vi "Plot_RoofShape.vi"() -> ()   [LabVIEW 2014]
uses:
  Anemometry/Anemometry Sub Vis/Controls/Server_Comms.ctl
  Anemometry/Anemometry Sub Vis/File/Setup_Filetype.ctl
  <vilib>/printing/EasyPrintingControls.llb/report_type.ctl
  <vilib>/printing/EasyPrintingControls.llb/layout_options.ctl
  <vilib>/printing/EasyPrintingControls.llb/orientation.ctl
  <vilib>/printing/EasyPrintingControls.llb/panel_scaling_for_page.ctl
  <vilib>/printing/EasyPrintingControls.llb/margins.ctl
  <vilib>/printing/EasyPrintingControls.llb/margin_values.ctl
  <vilib>/printing/EasyPrintingControls.llb/measurement_system.ctl
  <vilib>/printing/EasyPrintingControls.llb/printer_options.ctl
  <vilib>/printing/EasyPrintingControls.llb/printing_method.ctl
  <vilib>/printing/EasyPrintingControls.llb/color_or_monochrome.ctl
  <vilib>/printing/EasyPrintingControls.llb/page_header_options.ctl
  <vilib>/printing/EasyPrintingControls.llb/page_headers.ctl
  <vilib>/printing/EasyPrintingControls.llb/page_header_content_options.ctl
  <vilib>/printing/EasyPrintingControls.llb/custom_contents_options.ctl
  <vilib>/printing/EasyPrintingControls.llb/list_which_controls.ctl
  Anemometry/Anemometry Sub Vis/Globals/Preference_global.vi
  <vilib>/printing/EasyPrinting.llb/Easy Print VI Panel or Documentation (path).vi
  <vilib>/Utility/NIReport.llb/NI_ReportGenerationCore.lvlib
  <vilib>/Utility/SMTP/NI_SMTPEmail.lvlib
panel:
  in  "Units Selector":u16(ring) items=["Metric", "English"]
  in  "Tab Control":T1(tab)=enum."Real-Time"
  in  "History\n(mins)":dbl=2.0 format="%.1f"
  in  "Mode":T2(ring)=enum."Display data over specified period:"
  in  "Throwback\n(mins)":dbl format="%.1f"
  out "LastUpdated":string="Wed, Jul 29, 2015 at 4:31 PM"
  out "Plot 1":cluster{"Times":dbl[], "Output array":dbl[]}[](graph)
  in  "Search 4":string="tunnel3:avstat" caption="Search:"
  in  "Selector 4":i32[](listbox)=[0, 1, 2, 3, 4, 5, 6, 7, 8, 9]
  in  "Save 1":bool
  in  "Precision":i32=2
  in  "Selector 5":i32[](listbox)=[0, 1, 2, 3, 4, 5, 6, 7]
  in  "Search 5":string="tunnel3:Avstat" caption="Search:"
  in  "Selector 6":i32[](listbox)=[0, 1, 2, 3, 4, 5, 6, 7]
  in  "Search 6":string="rangeroof" caption="Search:"
  out "x < y?":bool=TRUE caption="In Range"
  in  "Save 3":bool
  out "Plot 3":cluster{"Times":dbl[], "Output array":dbl[]}[](graph)=[{"Times"=[1.0, 2.0, 3.0, 4.0, 5.0, 6.0, 7.0, 8.0], "Output array"=[0.0, 0.0, 0.0, 4.0, 9.0, 11.0, 13.0, 3.0]}, {"Times"=[1.0, 2.0, 3.0, 4.0, 5.0, 6.0, 7.0, 8.0], "Output array"=[-0.002410980854964788, -0.0029939228778896234, -0.002989543855604076, -0.000737475319318735, -0.0014917557433837283, -0.0018513430195620808, -0.0021749907541396205, -0.0013073221118501653]}, {"Times"=[8.0, 1.0], "Output array"=[-0.000737475319318735, -0.000737475319318735]}, {"Times"=[8.0, 1.0], "Output array"=[-0.0029939228778896234, -0.0029939228778896234]}]
  out "Roof Height":dbl[](array[numeric])=[0.0, 0.0, 0.0, 4.0, 9.0, 11.0, 13.0, 3.0] caption="Roof Height (cm)"
  out "Failed recipients":string[](array[string])
  in  "Recipients":string[](array[string])=["ttech@cppwind.com"]
  in  "mail server":string="post.cppwind.local"
  in  "print?":bool
  in  "email?":bool
  in  "Save plot number":T3(ring)
  out "Plot 1 Chs":string[](array[string])=["Tunnel3:AvStat:P1", "Tunnel3:AvStat:P2", "Tunnel3:AvStat:P3", "Tunnel3:AvStat:P4", "Tunnel3:AvStat:P5", "Tunnel3:AvStat:P6", "Tunnel3:AvStat:P7", "Tunnel3:AvStat:P8", "Tunnel3:AvStat:+PFan", "Tunnel3:AvStat:P0"]
  out "Plot 2 Chs":string[](array[string])=["Tunnel3:AvStat:P1", "Tunnel3:AvStat:P2", "Tunnel3:AvStat:P3", "Tunnel3:AvStat:P4", "Tunnel3:AvStat:P5", "Tunnel3:AvStat:P6", "Tunnel3:AvStat:P7", "Tunnel3:AvStat:P8"]
  out "Plot 3 Chs":string[](array[string])=["Tunnel3:RangeRoof:1", "Tunnel3:RangeRoof:2", "Tunnel3:RangeRoof:3", "Tunnel3:RangeRoof:4", "Tunnel3:RangeRoof:5", "Tunnel3:RangeRoof:6", "Tunnel3:RangeRoof:7", "Tunnel3:RangeRoof:8"]
  in  "Save 2":bool
  out "Plot 2":cluster{dbl[], "Output array":dbl[]}(graph)={[1.0, 2.0, 3.0, 4.0, 5.0, 6.0, 7.0, 8.0], "Output array"=[-0.002410980854964788, -0.0029939228778896234, -0.002989543855604076, -0.000737475319318735, -0.0014917557433837283, -0.0018513430195620808, -0.0021749907541396205, -0.0013073221118501653]}
  in  "stop":bool=TRUE
  # "Select Pressure Measurement"
  # "Select Height Measurement"
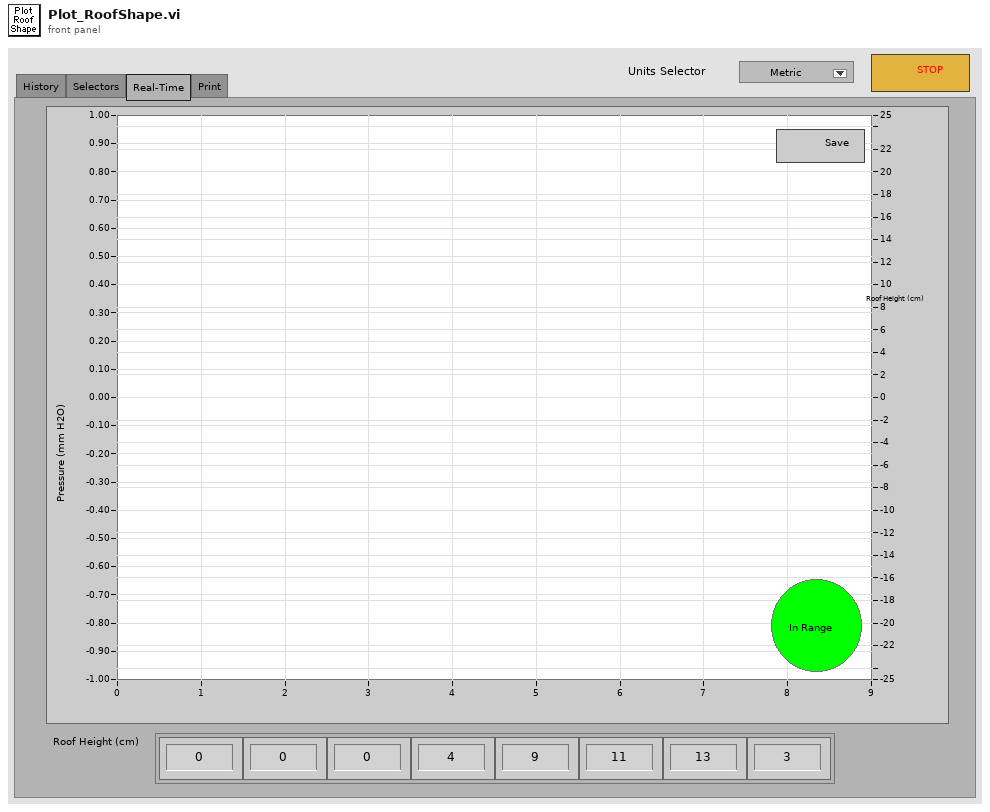
[diagram p1: front panel]
types:
  T1 = enum32{"History", "Selectors", "Real-Time", "Print"}
  T2 = enum16{"Display full time history", "Display data over specified period:"}
  T3 = enum16{"Save Plot 1", "Save Plot 2", "Save Plot 3"}
  T4 = typedef "Server_Comms.ctl" = enum16{"Server Link Healthy", "Do Not Link To Server"}
  T5 = typedef "Setup_Filetype.ctl" = enum16{"Measurement Setups", "Calibration Setups", "General", "Results File Plotter Setups", "Speed Calib Tweaks"}
  T6 = cluster{"path":path, "data":string, "binary":bool, "MIME content-type \n(application/octet-stream)":string}
  T7 = typedef "NI_ReportGenerationCore.lvlib/custom_contents_options.ctl" = cluster{"include VI connector and icon":bool, "include VI description":bool, "include front panel":bool, "surround front panel with border":bool, "list of controls options":cluster{"include list of controls":bool, "list which controls?":T8, "include control descriptions?":bool, "include control data types?":bool}, "block diagram options":cluster{"include block diagram":bool, "hidden frames":bool, "ordered (repeat from higher level if nested)":bool}, "include VI hierarchy":bool, "include list of subVIs":bool, "include VI history":bool, "include Express VI configuration information":bool}
  T8 = typedef "NI_ReportGenerationCore.lvlib/list_which_controls.ctl" = u16
  T9 = typedef "NI_ReportGenerationCore.lvlib/layout_options.ctl" = cluster{"orientation (unchanged)":T10, "panel scaling for page (unchanged)":T11, "margins":T12, "printer options":T15, "page header options":T18}
  T10 = typedef "NI_ReportGenerationCore.lvlib/orientation.ctl" = u16
  T11 = typedef "NI_ReportGenerationCore.lvlib/panel_scaling_for_page.ctl" = u16
  T12 = typedef "NI_ReportGenerationCore.lvlib/margins.ctl" = cluster{"override VI margins (false)":bool, "margins (1.00)":T13, "measurement system (default)":T14}
  T13 = typedef "NI_ReportGenerationCore.lvlib/margin_values.ctl" = cluster{"top":dbl, "left":dbl, "right":dbl, "bottom":dbl}
  T14 = typedef "NI_ReportGenerationCore.lvlib/measurement_system.ctl" = u16
  T15 = typedef "NI_ReportGenerationCore.lvlib/printer_options.ctl" = cluster{"destination printer name (current)":string, "printing method (unchanged)":T16, "color or monochrome (unchanged)":T17}
  T16 = typedef "NI_ReportGenerationCore.lvlib/printing_method.ctl" = u16
  T17 = typedef "NI_ReportGenerationCore.lvlib/color_or_monochrome.ctl" = u16
  T18 = typedef "NI_ReportGenerationCore.lvlib/page_header_options.ctl" = cluster{"page headers (unchanged)":T19, "page header content options":T20}
  T19 = typedef "NI_ReportGenerationCore.lvlib/page_headers.ctl" = u16
  T20 = typedef "NI_ReportGenerationCore.lvlib/page_header_content_options.ctl" = cluster{"Include VI Name":bool, "Include VI Path":bool, "Include Last Modification Date":bool, "Include Date Printed":bool, "Include Page Number":bool, "Include VI Icon":bool}
  T21 = typedef "NI_ReportGenerationCore.lvlib/report_type.ctl" = u16
  T22 = cluster{"path":path, "data":string, "binary":bool, "MIME content-type \n(application/octet-stream)":string}[]
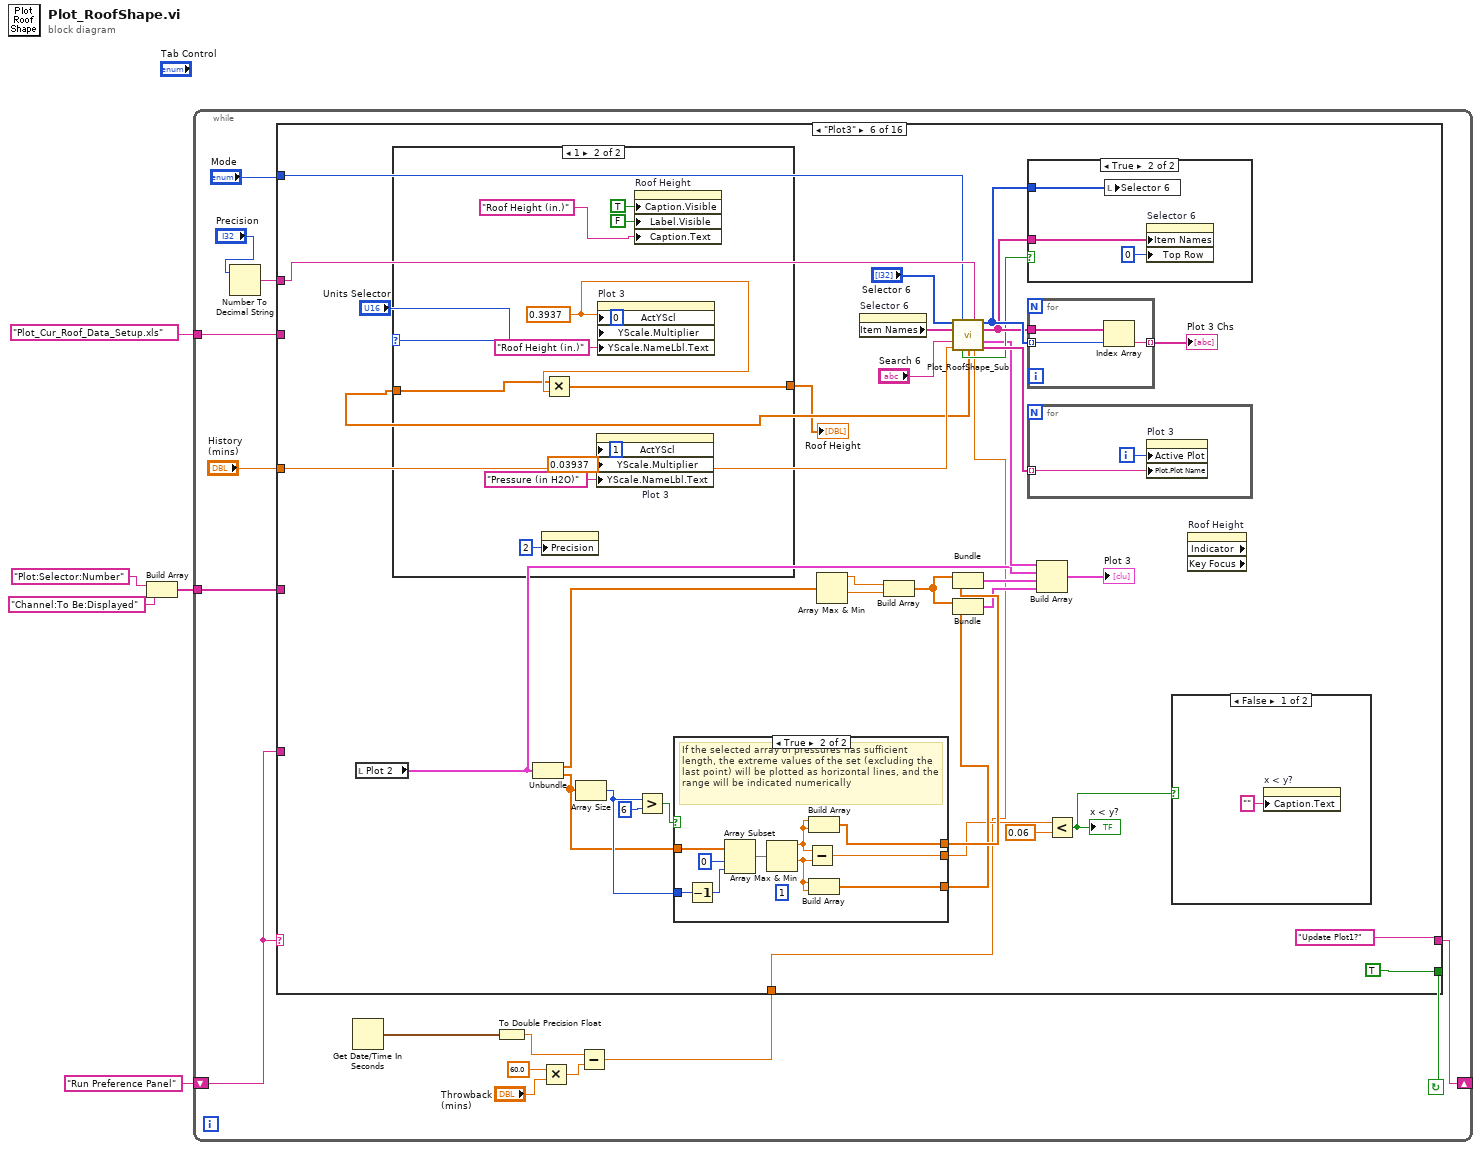
[diagram p0: block diagram]
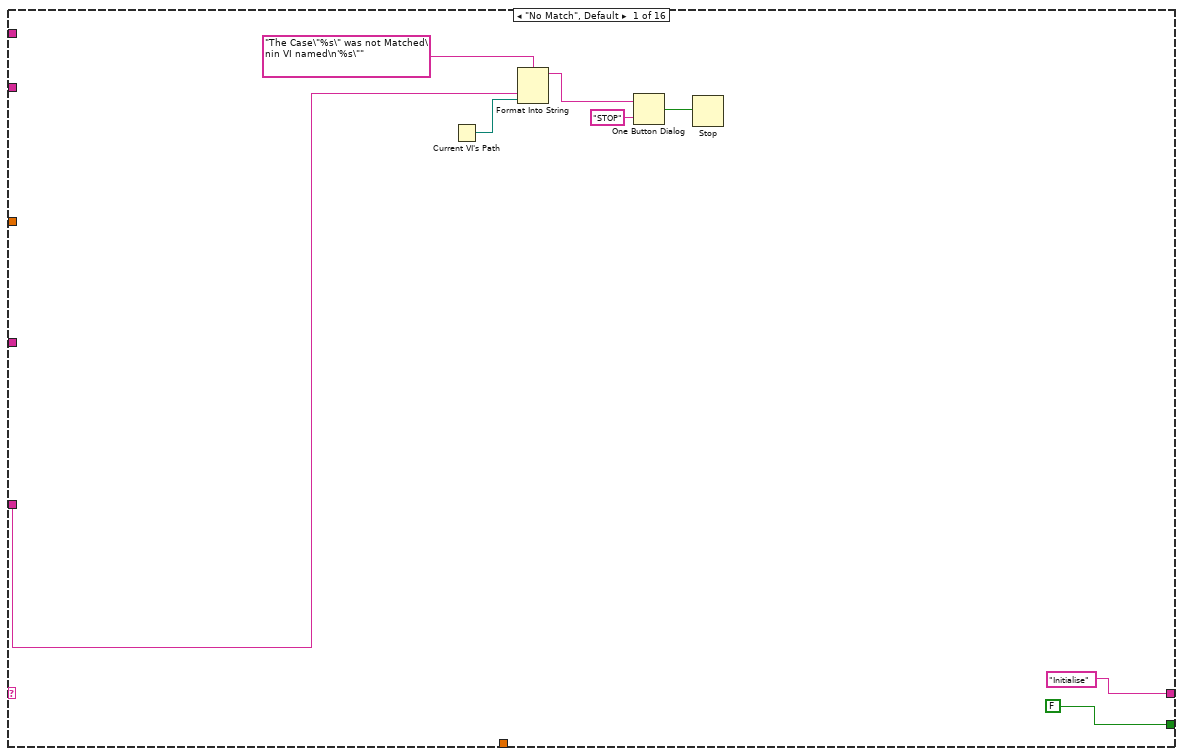
[diagram p2: hidden frame]
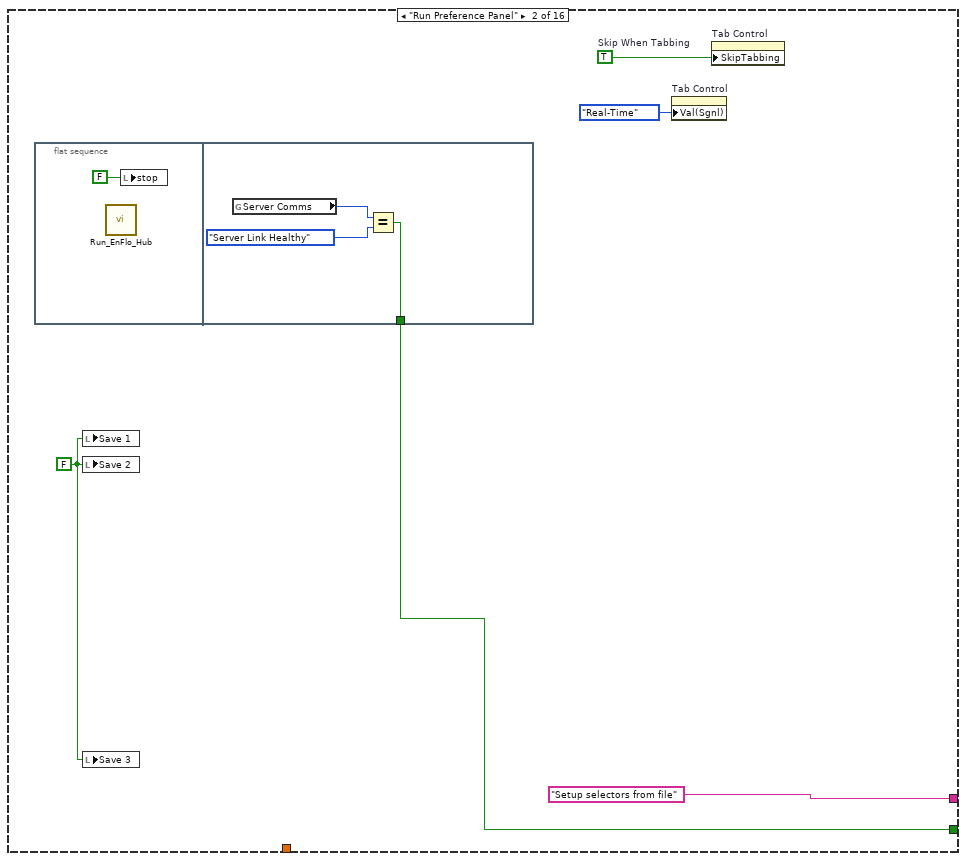
[diagram p3: hidden frame]
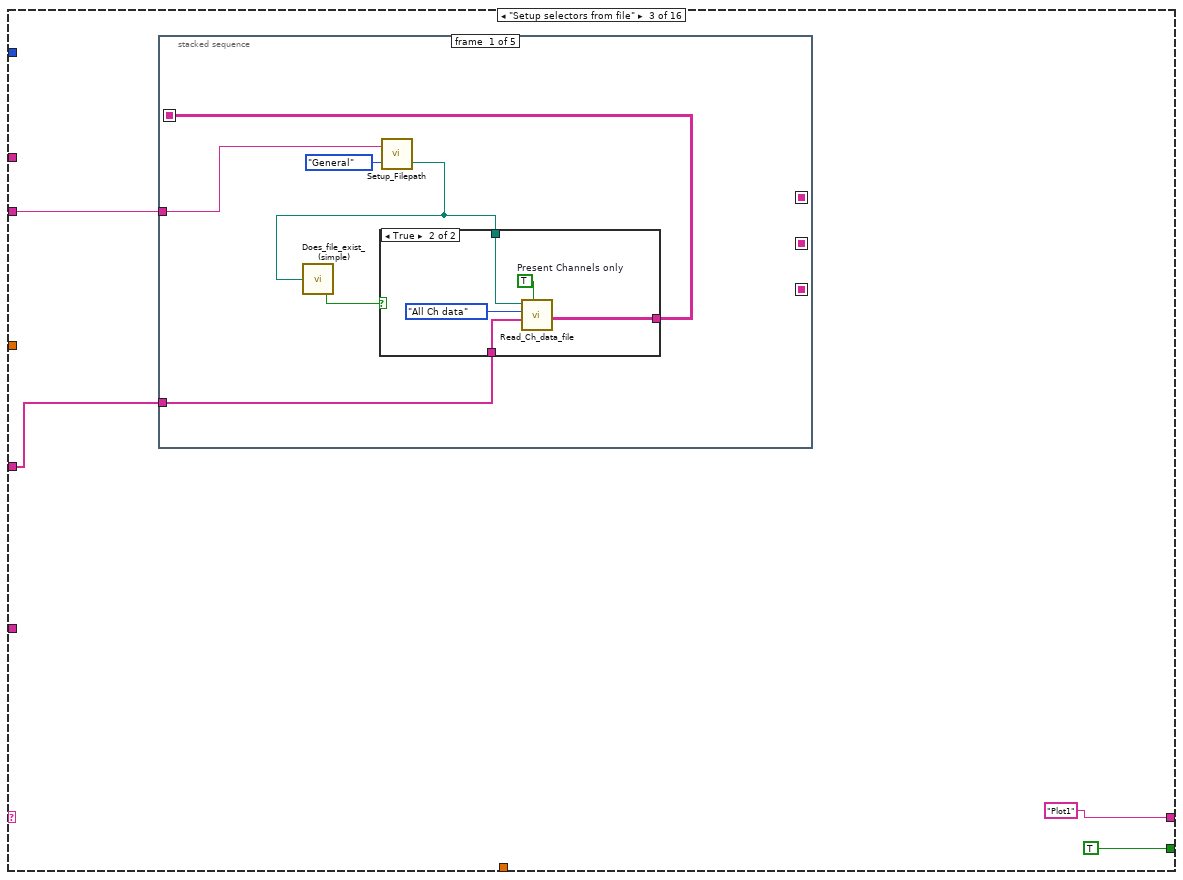
[diagram p4: hidden frame]
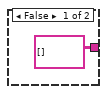
[diagram p5: hidden frame]
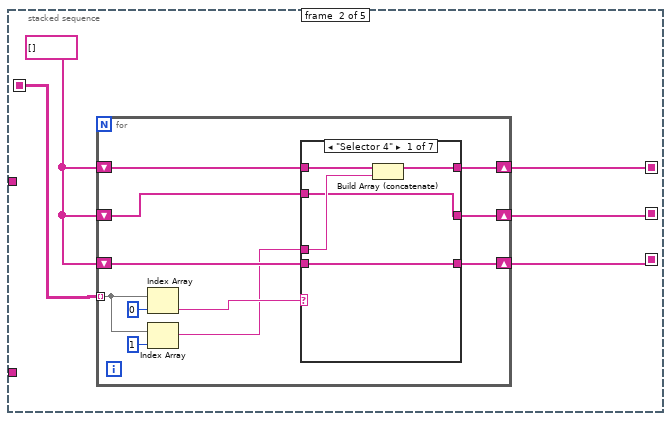
[diagram p6: hidden frame]
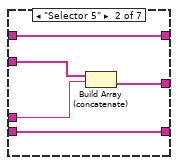
[diagram p7: hidden frame]
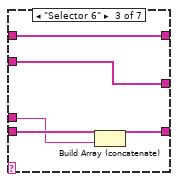
[diagram p8: hidden frame]
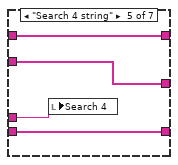
[diagram p10: hidden frame]
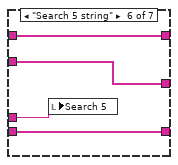
[diagram p11: hidden frame]
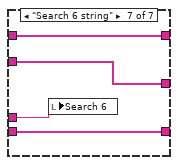
[diagram p12: hidden frame]
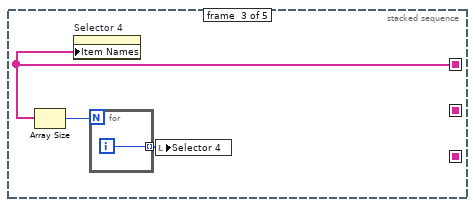
[diagram p13: hidden frame]
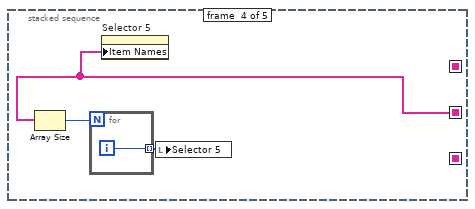
[diagram p14: hidden frame]
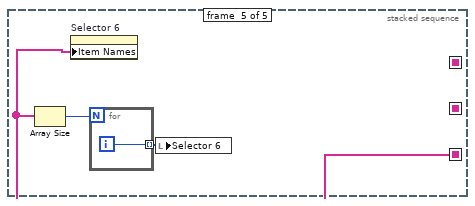
[diagram p15: hidden frame]
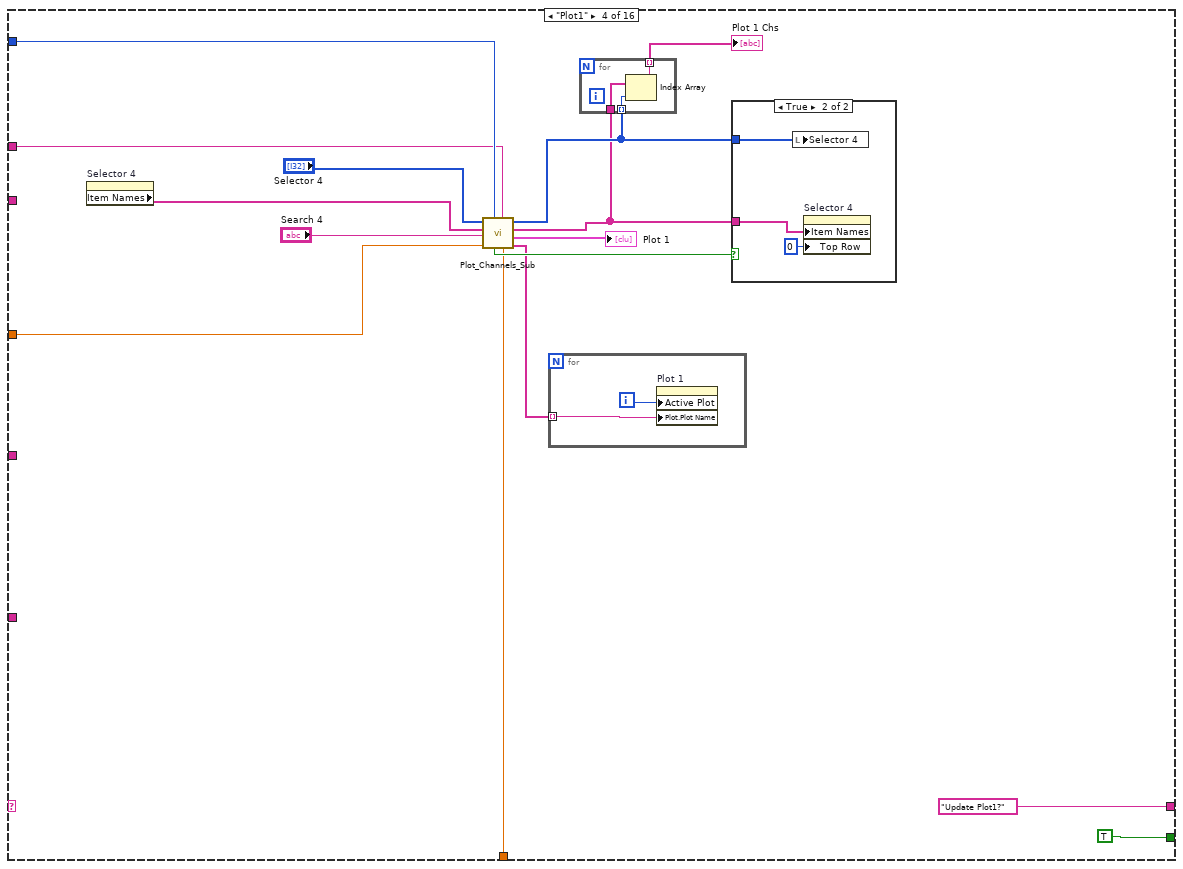
[diagram p16: hidden frame]
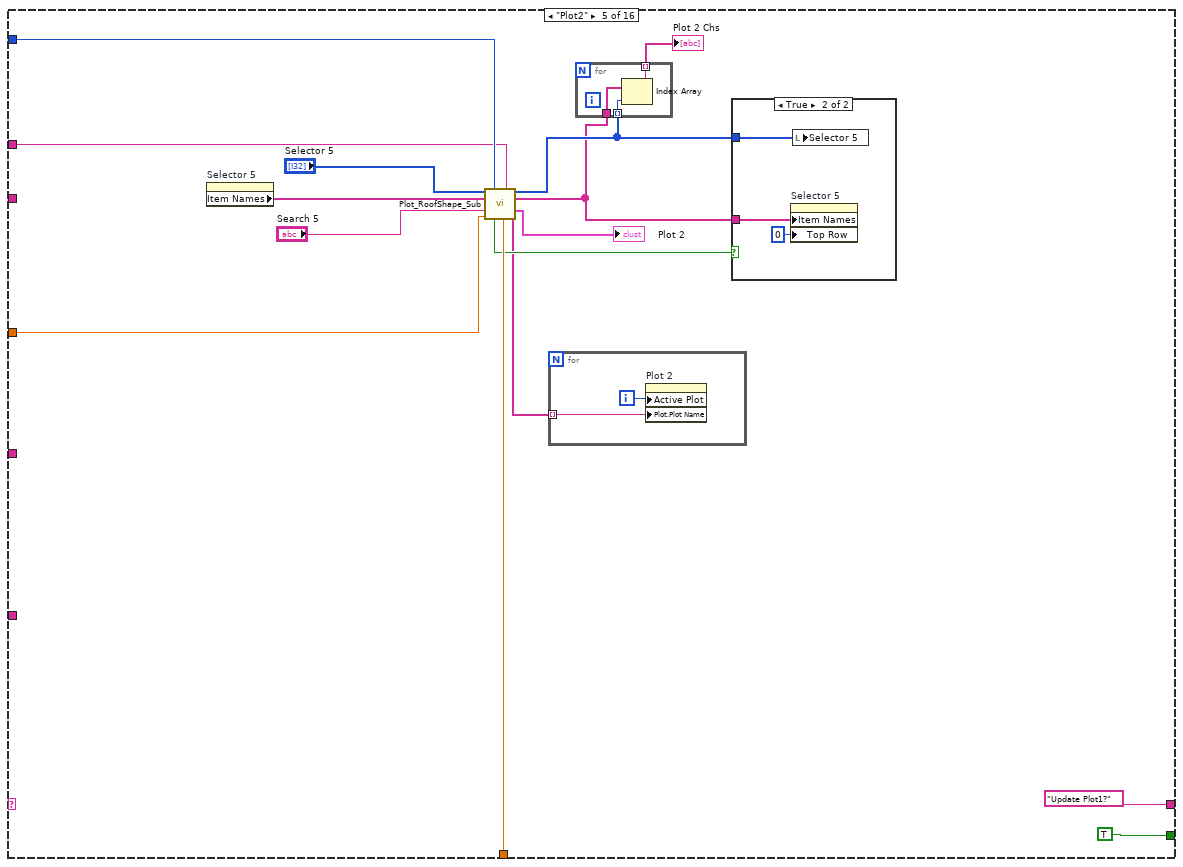
[diagram p18: hidden frame]
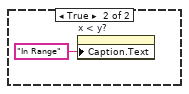
[diagram p20: hidden frame]
diagram:
  n1 = Build Array("Plot:Selector:Number", "Channel:To Be:Displayed") -> (w2:string[])
  n2 = while {
    shift-left: "Run Preference Panel" -> [w18]
    shift-right: [w19] -> _
    tunnel: w2 -> [w15]
    tunnel: "Plot_Cur_Roof_Data_Setup.xls" -> [w14]
    stop <- w20 continue-if-true
    n3 = Number To Decimal String(number="Precision") -> (decimal integer string=w12:string)  [unwired: 1 out]
    n4 = Get Date/Time In Seconds() -> (seconds since 1Jan1904=w11:timestamp)
    n5 = To Double Precision Float(number=w11) -> (double precision float=w7:dbl)
    n6 = Multiply(x=60.0, y="Throwback\n(mins)") -> (x*y=w8:dbl)
    n7 = Subtract(x=w7, y=w8) -> (x-y=w6:dbl)
    n8 = case shown="\"Plot3\"" w18 {
      tunnel: [FALSE w32 TRUE TRUE TRUE TRUE TRUE TRUE TRUE TRUE w371 TRUE TRUE TRUE TRUE w473] -> w20
      tunnel: ["Initialise" "Setup selectors from file" "Plot1" "Update Plot1?" "Update Plot1?" "Update Plot1?" w239 w260 w280 w300 w372 w431 "Email" ("t") "CleanUp" ("t") "What to do next?" "Update Plot1?" ("t")] -> w19
      tunnel: w18 -> [w23 _ _ _ _ _ _ _ _ _ _ _ _ _ _ _]
      tunnel: "Mode" -> [_ _ _ w119 w140 w180 _ _ _ _ _ _ _ _ _ _]
      tunnel: "History\n(mins)" -> [_ _ _ w118 w145 w189 _ _ _ _ _ _ _ _ _ _]
      tunnel: w15 -> [_ _ w38 _ _ _ _ _ _ _ _ _ _ _ _ w477]
      tunnel: w14 -> [_ _ w39 _ _ _ _ _ _ _ _ _ _ _ _ w476]
      tunnel: w12 -> [_ _ _ w113 w135 w185 _ _ _ _ _ _ _ _ _ _]
      tunnel: w6 -> [_ _ _ w112 w146 w162 _ _ _ _ _ _ _ _ _ _]
      frame "No Match", Default {
        n9 = Current VI's Path() -> (path=w22:path)
        n10 = Format Into String(format string="The Case\"%s\" was not Matched\nin VI named\n'%s\"" ("Format String"), w23, w22) -> (resulting string=w26:string)  [unwired: 2 in, 1 out]
        n11 = One Button Dialog(message=w26, button name ("OK")="STOP") -> (true=w24:bool)
        n12 = Stop(stop? (T)=w24) -> ()
      }
      frame "Run Preference Panel" {
        w29 = TRUE  # Skip When Tabbing
        w31 = FALSE ("Save 1")
        n13 = flat-sequence {
          tunnel: [w35] -> w32
          frame #0 {
            n14 = call "Run_EnFlo_Hub.vi"() -> ()  [unwired: 8 out]
            n15 = local write "stop"(FALSE ("stop")) -> ()
          }
          frame #1 {
            n16 = global read "Preference_global.vi" "Server Comms"() -> (w36:T4)
            n17 = Equal?(x=w36, y=Server_Comms."Server Link Healthy" ("Server Comms")) -> (x = y?=w35:bool)
          }
        }
        n18 = local write "Save 1"(w31) -> ()
        n19 = local write "Save 2"(w31) -> ()
        n20 = local write "Save 3"(w31) -> ()
        n21 = property on="Tab Control" class="TabCtl (strict)"("Val(Sgnl)"=T1."Real-Time" ("Value (Signaling)")) -> ()  [unwired: 2 in, 2 out]
        n22 = property on="Tab Control" class="TabCtl (strict)"("SkipTabbing"=w29) -> ()  [unwired: 2 in, 2 out]
      }
      frame "Setup selectors from file" {
        n23 = stacked-sequence {
          seq-local: [w45 _ _ _ _] -> [_ w58 _ _ _]
          seq-local: [_ w56 _ _ _] -> [_ _ w102 _ _]
          seq-local: [_ w54 _ _ _] -> [_ _ _ w104 _]
          seq-local: [_ w55 _ _ _] -> [_ _ _ _ w108]
          tunnel: w39 -> [w44 _ _ _ _]
          tunnel: w38 -> [w46 _ _ _ _]
          frame #0 {
            n24 = call "Setup_Filepath.vi"("Setup File Type"=Setup_Filetype."General", "Filename in"=w44) -> ("Filename Out"=w43:path)  [unwired: 1 out]
            n25 = call "Does_file_exist_(simple).vi"("Pathname"=w43) -> ("exists?"=w47:bool)
            n26 = case shown="True" w47 {
              tunnel: w43 -> [_ w53]
              tunnel: w46 -> [_ w52]
              tunnel: [string[][] [] ("Channel Values") w49] -> w45
              frame False {
              }
              frame True {
                w51 = TRUE  # Present Channels only
                n27 = call "Read_Ch_data_file.vi"("Present Channels only"=w51, "Present Channels"=w52, "Output"=enum16{"All Ch data", "The last few rows"}."All Ch data", "Filename"=w53) -> ("Channel Values"=w49:string[][])  [unwired: 1 in, 4 out]
              }
            }
          }
          frame #1 {
            w57 = string[] []
            n28 = for {
              shift-right: [w64] -> w56
              shift-left: w57 -> [w65]
              tunnel: w58 -> [w66] mode=indexing
              shift-right: [w62] -> w54
              shift-left: w57 -> [w63]
              shift-right: [w60] -> w55
              shift-left: w57 -> [w61]
              n29 = Index Array(array=w66, index=0 ("Index")) -> (element=w68:string)
              n30 = Index Array(array=w66, index=1 ("Index")) -> (element=w59:string)
              n31 = case shown="\"Selector 4\"" w68 {
                tunnel: w65 -> [w74 w79 w80 w86 w90 w94 w98]
                tunnel: [w73 w79 w80 w86 w90 w94 w98] -> w64
                tunnel: w59 -> [w72 w76 w82 _ w88 w92 w96]
                tunnel: w63 -> [w71 w77 w81 w87 w91 w95 w99]
                tunnel: [w71 w75 w81 w87 w91 w95 w99] -> w62
                tunnel: w61 -> [w70 w78 w84 w85 w89 w93 w97]
                tunnel: [w70 w78 w83 w85 w89 w93 w97] -> w60
                frame "Selector 4" {
                  n32 = Build Array (concatenate)(w74, w72) -> (w73:string[])
                }
                frame "Selector 5" {
                  n33 = Build Array (concatenate)(w77, w76) -> (w75:string[])
                }
                frame "Selector 6" {
                  n34 = Build Array (concatenate)(w84, w82) -> (w83:string[])
                }
                frame "No Match", Default {
                }
                frame "Search 4 string" {
                  n35 = local write "Search 4"(w88) -> ()
                }
                frame "Search 5 string" {
                  n36 = local write "Search 5"(w92) -> ()
                }
                frame "Search 6 string" {
                  n37 = local write "Search 6"(w96) -> ()
                }
              }
            }
          }
          frame #2 {
            n38 = Array Size(array=w102) -> (size(s)=w101:i32)
            n39 = property on="Selector 4" class="LstBox (strict)"("Item Names"=w102) -> ()  [unwired: 2 in, 2 out]
            n40 = for {
              N: w101 -> [_]
              tunnel: [w103] -> w100 mode=indexing
              i -> [w103]
            }
            n41 = local write "Selector 4"(w100) -> ()
          }
          frame #3 {
            n42 = Array Size(array=w104) -> (size(s)=w106:i32)
            n43 = for {
              N: w106 -> [_]
              tunnel: [w107] -> w105 mode=indexing
              i -> [w107]
            }
            n44 = property on="Selector 5" class="LstBox (strict)"("Item Names"=w104) -> ()  [unwired: 2 in, 2 out]
            n45 = local write "Selector 5"(w105) -> ()
          }
          frame #4 {
            n46 = Array Size(array=w108) -> (size(s)=w110:i32)
            n47 = property on="Selector 6" class="LstBox (strict)"("Item Names"=w108) -> ()  [unwired: 2 in, 2 out]
            n48 = for {
              N: w110 -> [_]
              tunnel: [w111] -> w109 mode=indexing
              i -> [w111]
            }
            n49 = local write "Selector 6"(w109) -> ()
          }
        }
      }
      frame "Plot1" {
        n50 = property on="Selector 4" class="LstBox (strict)"() -> ("Item Names"=w121:string[])  [unwired: 2 in, 2 out]
        n51 = call "Plot_Channels_Sub.vi"("End Time"=w112, "precision"=w113, "Mode"=w119, "History (min)"=w118, "Search String"="Search 4", "Selector List In"=w121, "Selector array In"="Selector 4") -> ("Plot Legend"=w117:string[], "Plot"=→"Plot 1":cluster{"Times":dbl[], "Output array":dbl[]}[], "Selector List Out"=w115:string[], "Selector array Out"=w116:i32[], "Selector Changed?"=w123:bool)
        n52 = for {
          tunnel: w117 -> [w130] mode=indexing
          i -> [w131]
          n53 = property on="Plot 1" class="XYGraph (strict)"("Active Plot"=w131, "Plot.Plot Name"=w130) -> ()  [unwired: 2 in, 2 out]
        }
        n54 = for {
          tunnel: w116 -> [w129] mode=indexing
          tunnel: w115 -> [w128]
          tunnel: [w127] -> w114 mode=indexing
          n55 = Index Array(array=w128, index=w129) -> (element=w127:string)
        }
        "Plot 1 Chs" <- w114
        n56 = case shown="True" w123 {
          tunnel: w115 -> [_ w134]
          tunnel: w116 -> [_ w133]
          frame False {
          }
          frame True {
            n57 = local write "Selector 4"(w133) -> ()
            n58 = property on="Selector 4" class="LstBox (strict)"("Item Names"=w134, "Top Row"=0) -> ()  [unwired: 2 in, 2 out]
          }
        }
      }
      frame "Plot2" {
        n59 = property on="Selector 5" class="LstBox (strict)"() -> ("Item Names"=w142:string[])  [unwired: 2 in, 2 out]
        n60 = call "Plot_RoofShape_Sub.vi"("Selector array In"="Selector 5", "Mode"=w140, "precision"=w135, "Selector List In"=w142, "Search String"="Search 5", "History (min)"=w145, "End Time"=w146) -> ("Selector array Out"=w139:i32[], "Selector List Out"=w138:string[], "Plot"=→"Plot 2":cluster{dbl[], "Output array":dbl[]}, "Selector Changed?"=w143:bool, "Plot Legend"=w136:string[])  [unwired: 2 in, 2 out]
        n61 = for {
          tunnel: w136 -> [w153] mode=indexing
          i -> [w154]
          n62 = property on="Plot 2" class="XYGraph (strict)"("Active Plot"=w154, "Plot.Plot Name"=w153) -> ()  [unwired: 2 in, 2 out]
        }
        n63 = for {
          tunnel: w139 -> [w152] mode=indexing
          tunnel: w138 -> [w151]
          tunnel: [w150] -> w147 mode=indexing
          n64 = Index Array(array=w151, index=w152) -> (element=w150:string)
        }
        "Plot 2 Chs" <- w147
        n65 = case shown="True" w143 {
          tunnel: w138 -> [_ w156]
          tunnel: w139 -> [_ w157]
          frame False {
          }
          frame True {
            n66 = property on="Selector 5" class="LstBox (strict)"("Item Names"=w156, "Top Row"=0) -> ()  [unwired: 2 in, 2 out]
            n67 = local write "Selector 5"(w157) -> ()
          }
        }
      }
      frame "Plot3" {
        n68 = local read "Plot 2"() -> (w167:cluster{dbl[], "Output array":dbl[]})
        n69 = Unbundle(w167) -> (w166:dbl[], "Output array"=w165:dbl[])
        n70 = Array Size(array=w165) -> (size(s)=w176:i32)
        n71 = Greater?(x=w176, y=6) -> (0:w175:bool)
        n72 = case shown="True" w175 {
          tunnel: w165 -> [_ w229]
          tunnel: w176 -> [_ w228]
          tunnel: [w219 w223] -> w172
          tunnel: [w219 w224] -> w170
          tunnel: [w218 w220] -> w164
          frame False {
            w218 = 0.0
            n73 = Build Array(w218, w218) -> (w219:dbl[])
          }
          frame True {
            (unwired) 1
            # "If the selected array of pressures has sufficient length, the extreme values of the set (excluding the last point) will be plotted as horizontal lines, and the range will be indicated numerically"
            n74 = Decrement(x=w228) -> (x-1=w227:i32)
            n75 = Array Subset(array=w229, index=0, length=w227) -> (w225:dbl[])
            n76 = Array Max & Min(array=w225) -> (max value=w222:dbl, min value=w221:dbl)  [unwired: 2 out]
            n77 = Subtract(x=w222, y=w221) -> (x-y=w220:dbl)
            n78 = Build Array(w222, w222) -> (w223:dbl[])
            n79 = Build Array(w221, w221) -> (w224:dbl[])
          }
        }
        n80 = Array Max & Min(array=w166) -> (max value=w173:dbl, min value=w174:dbl)  [unwired: 2 out]
        n81 = property on="Selector 6" class="LstBox (strict)"() -> ("Item Names"=w187:string[])  [unwired: 2 in, 2 out]
        n82 = Build Array(w173, w174) -> (w171:dbl[])
        n83 = call "Plot_RoofShape_Sub.vi"("Selector array In"="Selector 6", "Mode"=w180, "precision"=w185, "Selector List In"=w187, "Search String"="Search 6", "History (min)"=w189, "End Time"=w162) -> ("Selector array Out"=w184:i32[], "Selector List Out"=w183:string[], "Plot"=w179:cluster{dbl[], "Output array":dbl[]}, "Selector Changed?"=w181:bool, "Position Values"=w160:dbl[], "Plot Legend"=w182:string[])  [unwired: 2 in, 1 out]
        n84 = case shown="1" "Units Selector" {
          tunnel: w160 -> [w202 w214]
          tunnel: [w202 w213] -> w159
          frame 0, Default {
            n85 = property class="DigNum (strict)"("Precision"=u8 0 ("Display Format:Precision")) -> ()  [unwired: 2 in, 2 out]
            n86 = property on="Plot 3" class="XYGraph (strict)"("ActYScl"=1 ("Active Y Scale"), "YScale.Multiplier"=1.0 ("Y Scale.Offset and Multiplier:Multiplier"), "YScale.NameLbl.Text"="Pressure (mm H2O)" ("Y Scale.Name Label.Text")) -> ()  [unwired: 2 in, 2 out]
            n87 = property on="Plot 3" class="XYGraph (strict)"("ActYScl"=0 ("Active Y Scale"), "YScale.Multiplier"=1.0 ("Y Scale.Offset and Multiplier:Multiplier"), "YScale.NameLbl.Text"="Roof Height (cm)" ("Y Scale.Name Label.Text")) -> ()  [unwired: 2 in, 2 out]
            n88 = property on="Roof Height" class="Arr (strict)"("Caption.Visible"=TRUE, "Label.Visible"=FALSE, "Caption.Text"="Roof Height (cm)" ("Label.Text")) -> ()  [unwired: 2 in, 2 out]
          }
          frame 1 {
            w215 = 0.3937 ("Y Scale.Offset and Multiplier:Multiplier")
            n89 = property class="DigNum (strict)"("Precision"=u8 2 ("Display Format:Precision")) -> ()  [unwired: 2 in, 2 out]
            n90 = Multiply(x=w214, y=w215) -> (x*y=w213:dbl[])
            n91 = property on="Plot 3" class="XYGraph (strict)"("ActYScl"=1 ("Active Y Scale"), "YScale.Multiplier"=0.03937 ("Y Scale.Offset and Multiplier:Multiplier"), "YScale.NameLbl.Text"="Pressure (in H2O)" ("Y Scale.Name Label.Text")) -> ()  [unwired: 2 in, 2 out]
            n92 = property on="Plot 3" class="XYGraph (strict)"("ActYScl"=0 ("Active Y Scale"), "YScale.Multiplier"=w215, "YScale.NameLbl.Text"="Roof Height (in.)" ("Y Scale.Name Label.Text")) -> ()  [unwired: 2 in, 2 out]
            n93 = property on="Roof Height" class="Arr (strict)"("Caption.Visible"=TRUE, "Label.Visible"=FALSE, "Caption.Text"="Roof Height (in.)" ("Label.Text")) -> ()  [unwired: 2 in, 2 out]
          }
        }
        "Roof Height" <- w159
        n94 = Bundle(w171, w172) -> (w169:cluster{dbl[], dbl[]})  [unwired: 1 out]
        n95 = Bundle(w171, w170) -> (w168:cluster{dbl[], dbl[]})  [unwired: 1 out]
        n96 = case shown="True" w181 {
          tunnel: w183 -> [_ w236]
          tunnel: w184 -> [_ w237]
          frame False {
          }
          frame True {
            n97 = local write "Selector 6"(w237) -> ()
            n98 = property on="Selector 6" class="LstBox (strict)"("Item Names"=w236, "Top Row"=0) -> ()  [unwired: 2 in, 2 out]
          }
        }
        n99 = for {
          tunnel: w184 -> [w232] mode=indexing
          tunnel: w183 -> [w231]
          tunnel: [w230] -> w190 mode=indexing
          n100 = Index Array(array=w231, index=w232) -> (element=w230:string)
        }
        "Plot 3 Chs" <- w190
        n101 = for {
          tunnel: w182 -> [w233] mode=indexing
          i -> [w234]
          n102 = property on="Plot 3" class="XYGraph (strict)"("Active Plot"=w234, "Plot.Plot Name"=w233) -> ()  [unwired: 2 in, 2 out]
        }
        n103 = Build Array(w179, w167, w169, w168) -> (→"Plot 3":cluster{dbl[], "Output array":dbl[]}[])
        n104 = Less?(x=w164, y=0.06) -> (x < y?=w158:bool)
        "x < y?" <- w158
        n105 = case shown="False" w158 {
          frame False {
            n106 = property on="x < y?" class="Bool (strict)"("Caption.Text"="") -> ()  [unwired: 2 in, 2 out]
          }
          frame True {
            n107 = property on="x < y?" class="Bool (strict)"("Caption.Text"="In Range") -> ()  [unwired: 2 in, 2 out]
          }
        }
        n108 = property on="Roof Height" class="Arr (strict)" props=["Indicator", "Key Focus"]() -> ()  [unwired: 2 in, 4 out]
      }
      frame "Update Plot1?" {
        n109 = while {
          shift-right: [w257] -> w246
          shift-left: _ -> [w254]
          shift-right: [w256] -> w248
          shift-left: _ -> [w255]
          tunnel: [w255] -> w247
          tunnel: [w254] -> w245
          stop <- FALSE continue-if-true
          n110 = local read "Selector 4"() -> (w257:i32[])
          n111 = local read "Search 4"() -> (w256:string)
        }
        n112 = case shown="False" "Save 1" {
          tunnel: ["Update Plot2?" "Save Plot" ("t")] -> w238
          frame False {
          }
          frame True {
            n113 = local write "Save plot number"(T3."Save Plot 1" ("Save plot number")) -> ()
          }
        }
        n114 = Equal?(x=w246, y=w245) -> (x = y?=w243:bool)
        n115 = Equal?(x=w247, y=w248) -> (x = y?=w244:bool)
        n116 = And(x=w243, y=w244) -> (x .and. y?=w242:bool)
        n117 = Select(t=w238, s=w242, f="Plot1") -> (s? t:f=w239:string)
      }
      frame "Update Plot2?" {
        n118 = while {
          shift-right: [w277] -> w266
          shift-left: _ -> [w274]
          shift-right: [w276] -> w268
          shift-left: _ -> [w275]
          tunnel: [w275] -> w267
          tunnel: [w274] -> w265
          stop <- FALSE continue-if-true
          n119 = local read "Selector 5"() -> (w277:i32[])
          n120 = local read "Search 5"() -> (w276:string)
        }
        n121 = case shown="False" "Save 2" {
          tunnel: ["Update Plot3?" "Save Plot" ("t")] -> w258
          frame False {
          }
          frame True {
            n122 = local write "Save plot number"(T3."Save Plot 2" ("Save plot number")) -> ()
          }
        }
        n123 = Equal?(x=w266, y=w265) -> (x = y?=w263:bool)
        n124 = Equal?(x=w267, y=w268) -> (x = y?=w264:bool)
        n125 = And(x=w263, y=w264) -> (x .and. y?=w262:bool)
        n126 = Select(t=w258, s=w262, f="Plot2") -> (s? t:f=w260:string)
      }
      frame "Update Plot3?" {
        n127 = while {
          shift-right: [w297] -> w286
          shift-left: _ -> [w294]
          shift-right: [w296] -> w288
          shift-left: _ -> [w295]
          tunnel: [w295] -> w287
          tunnel: [w294] -> w285
          stop <- FALSE continue-if-true
          n128 = local read "Selector 6"() -> (w297:i32[])
          n129 = local read "Search 6"() -> (w296:string)
        }
        n130 = case shown="False" "Save 3" {
          tunnel: ["What to do next?" "Save Plot" ("t")] -> w278
          frame False {
          }
          frame True {
            n131 = local write "Save plot number"(T3."Save Plot 3" ("Save plot number")) -> ()
          }
        }
        n132 = Equal?(x=w286, y=w285) -> (x = y?=w283:bool)
        n133 = Equal?(x=w287, y=w288) -> (x = y?=w284:bool)
        n134 = And(x=w283, y=w284) -> (x .and. y?=w282:bool)
        n135 = Select(t=w278, s=w282, f="Plot3") -> (s? t:f=w280:string)
      }
      frame "What to do next?" {
        n136 = Wait (ms)(milliseconds to wait=u32 300) -> ()  [unwired: 1 out]
        n137 = while {
          shift-right: [w335] -> _
          shift-left: _ -> [w334]
          shift-right: [w333] -> _
          shift-left: _ -> [w332]
          shift-right: [w325] -> _
          shift-left: _ -> [w324]
          tunnel: [w327] -> w299
          shift-right: [w321] -> w306
          shift-left: _ -> [w322]
          stop <- FALSE continue-if-true
          n138 = local read "History\n(mins)"() -> (w335:dbl)
          n139 = local read "Mode"() -> (w333:T2)
          n140 = Equal?(x=w335, y=w334) -> (x = y?=w331:bool)
          n141 = Equal?(x=w332, y=w333) -> (x = y?=w330:bool)
          n142 = And(x=w331, y=w330) -> (x .and. y?=w329:bool)
          n143 = Select(t=w324, s=w329, f=0) -> (s? t:f=w326:i32)
          n144 = case shown="6" w326 {
            tunnel: ["Plot1" "Plot2" "Plot3" "Update Plot1?" "Update Plot1?" "Update Plot1?" "Update Plot1?"] -> w327
            tunnel: w326 -> [w338 w342 w346 w352 w358 w364 _]
            tunnel: [w337 w341 w345 w351 w357 w363 0] -> w325
            tunnel: w322 -> [w336 w340 w344 w349 w355 w360 w367]
            tunnel: [w336 w340 w344 w348 w354 w361 w366] -> w321
            frame 0, Default {
              n145 = Increment(x=w338) -> (x+1=w337:i32)
            }
            frame 1 {
              n146 = Increment(x=w342) -> (x+1=w341:i32)
            }
            frame 2 {
              n147 = Increment(x=w346) -> (x+1=w345:i32)
            }
            frame 3 {
              n148 = Add(x=w349, y=1) -> (x+y=w348:i32)
              n149 = Increment(x=w352) -> (x+1=w351:i32)
            }
            frame 4 {
              n150 = Add(x=w355, y=1) -> (x+y=w354:i32)
              n151 = Increment(x=w358) -> (x+1=w357:i32)
            }
            frame 5 {
              n152 = Add(x=w360, y=1) -> (x+y=w361:i32)
              n153 = Increment(x=w364) -> (x+1=w363:i32)
            }
            frame 6 {
              n154 = Add(x=w367, y=1) -> (x+y=w366:i32)
            }
          }
        }
        n155 = Get Date/Time String(date format (0)=enum16{"short", "long", "abbreviated"}."abbreviated") -> (date string=w312:string, time string=w313:string)  [unwired: 2 out]
        n156 = Concatenate Strings(w312, " at " ("Substring"), w313) -> (→"LastUpdated":string)
        n157 = Quotient & Remainder(x=w306, y=500) -> (x-y*floor(x/y)=w309:i32)  [unwired: 1 out]
        n158 = Equal To 0?(x=w309) -> (x = 0?=w307:bool)
        n159 = Or(x="stop", y=w307) -> (x .or. y?=w298:bool)
        n160 = Or(x="print?", y="email?") -> (x .or. y?=w301:bool)
        n161 = case shown="False" w301 {
          tunnel: [w318 "Output" ("t")] -> w300
          tunnel: w299 -> [w317 _]
          tunnel: w298 -> [w316 _]
          frame False {
            n162 = Select(t="Save Channel Names", s=w316, f=w317) -> (s? t:f=w318:string)
          }
          frame True {
          }
        }
      }
      frame "Save Plot" {
        n163 = stacked-sequence {
          seq-local: [w381 _] -> [_ w408]
          seq-local: [w376 _] -> [_ w410]
          seq-local: [w380 _] -> [_ w409]
          tunnel: ["What to do next?" _] -> w372
          tunnel: [TRUE _] -> w371
          frame #0 {
            n164 = case shown="\"Save Plot 3\"" "Save plot number" {
              tunnel: [w389 w390 w394] -> w386
              tunnel: [w388 w393 w396] -> w381
              frame "Save Plot 1" {
                n165 = local write "Save 1"(FALSE ("Save 1")) -> ()
                n166 = local read "Plot 1 Chs"() -> (w388:string[])
                n167 = local read "Plot 1"() -> (w389:cluster{"Times":dbl[], "Output array":dbl[]}[])
              }
              frame "Save Plot 2" {
                n168 = local read "Plot 2"() -> (w391:cluster{dbl[], "Output array":dbl[]})
                n169 = local write "Save 2"(FALSE ("Save 1")) -> ()
                n170 = local read "Plot 2 Chs"() -> (w393:string[])
                n171 = Build Array(w391) -> (w390:cluster{dbl[], "Output array":dbl[]}[])
              }
              frame "Save Plot 3" {
                n172 = local write "Save 3"(FALSE ("Save 1")) -> ()
                n173 = local read "Plot 3"() -> (w394:cluster{"Times":dbl[], "Output array":dbl[]}[])
                n174 = local read "Plot 3 Chs"() -> (w396:string[])
              }
            }
            n175 = Index Array(array=w386, index=0) -> (element=w384:cluster{"Times":dbl[], "Output array":dbl[]})
            n176 = Unbundle(w384) -> ("Times"=w374:dbl[])  [unwired: 1 out]
            n177 = Get Date/Time In Seconds() -> (seconds since 1Jan1904=w378:timestamp)
            n178 = for {
              tunnel: w386 -> [w398] mode=indexing
              tunnel: [w397] -> w380 mode=indexing
              n179 = Unbundle(w398) -> ("Output array"=w397:dbl[])  [unwired: 1 out]
            }
            n180 = To Double Precision Float(number=w378) -> (double precision float=w377:dbl)
            n181 = Multiply(x=w374, y=60.0) -> (x*y=w375:dbl[])
            n182 = Add(x=w377, y=w375) -> (x+y=w376:dbl[])
          }
          frame #1 {
            w403 = FALSE  # append to file? (new file:F)
            n183 = for {
              tunnel: w409 -> [w427]
              tunnel: w410 -> [w421] mode=indexing
              tunnel: [w423] -> w402 mode=indexing
              i -> [w426]
              n184 = Number To Decimal String(number=w421) -> (decimal integer string=w422:string)  [unwired: 1 out]
              n185 = Index Array(array=w427, index (col)=w426) -> (element=w425:dbl[])  [unwired: 1 in]
              n186 = Get Date/Time String(seconds (now)=w421) -> (date string=w420:string, time string=w419:string)  [unwired: 2 out]
              n187 = for {
                tunnel: w425 -> [w429] mode=indexing
                tunnel: [w428] -> w424 mode=indexing
                n188 = call "Number_2_string.vi"("number"=w429) -> ("String"=w428:string)  [unwired: 1 in]
              }
              n189 = Build Array (concatenate)(w420, w419, w422, w424) -> (w423:string[])
            }
            n190 = Build Array (concatenate)("Date::", "Centre:Time:", "Seconds:Since:1st Jan 1904", w408) -> (w401:string[])
            n191 = call "Ch_names_to_rows.vi"("Channel Names"=w401) -> ("3 Row names"=w407:string[][])
            n192 = File Dialog(7:"Please choose file name" ("prompt")) -> (3:w415:path)  [unwired: 1 in, 8 out]
            n193 = Build Array (concatenate)(w407, w402) -> (w405:string[][])
            n194 = Strip Path(path=w415) -> (stripped path=w412:path, name=w414:string)
            n195 = call "Add_filename_suffix.vi"("Filename"=w414, "Suffix to add"=".xls") -> ("Filename out"=w411:string)  [unwired: 3 out]
            n196 = Array To Spreadsheet String(array=w405, 3:"%s" ("format string")) -> (spreadsheet string=w404:string)  [unwired: 1 out]
            n197 = Build Path(base path=w412, name or relative path=w411) -> (appended path=w400:path)
            n198 = call "Write_File_Simple.vi"("append to file? (new file:F)"=w403, "character string"=w404, "file path"=w400) -> ()  [unwired: 2 out]
          }
        }
      }
      frame "Output" {
        n199 = property on="Tab Control" class="TabCtl (strict)"("Val(Sgnl)"=T1."Real-Time" ("Value (Signaling)")) -> ()  [unwired: 2 in, 2 out]
        n200 = local read "print?"() -> (w432:bool)
        n201 = Select(t="Print", s=w432, f="Email") -> (s? t:f=w431:string)
      }
      frame "Print" {
        w441 = T7 {"include VI connector and icon"=FALSE, "include VI description"=FALSE, "include front panel"=FALSE, "surround front panel with border"=FALSE, "list of controls options"={"include list of controls"=FALSE, "list which controls?"=0, "include control descriptions?"=FALSE, "include control data types?"=FALSE}, "block diagram options"={"include block diagram"=FALSE, "hidden frames"=FALSE, "ordered (repeat from higher level if nested)"=FALSE}, "include VI hierarchy"=FALSE, "include list of subVIs"=FALSE, "include VI history"=FALSE, "include Express VI configuration information"=FALSE}  # custom contents options
        w440 = T9 {"orientation (unchanged)"=0, "panel scaling for page (unchanged)"=0, "margins"={"override VI margins (false)"=FALSE, "margins (1.00)"={"top"=1.0, "left"=1.0, "right"=1.0, "bottom"=1.0}, "measurement system (default)"=0}, "printer options"={"destination printer name (current)"="", "printing method (unchanged)"=0, "color or monochrome (unchanged)"=0}, "page header options"={"page headers (unchanged)"=1, "page header content options"={"Include VI Name"=FALSE, "Include VI Path"=FALSE, "Include Last Modification Date"=FALSE, "Include Date Printed"=TRUE, "Include Page Number"=FALSE, "Include VI Icon"=FALSE}}}  # layout options
        w439 = T21 0 items=["Quick Print", "Standard Report", "HTML", "Word", "Excel"] ("report type (Quick Print)")
        n202 = Current VI's Path() -> (path=w438:path)
        n203 = call-poly <vilib>:"Easy Print VI Panel or Documentation.vi"("custom contents options"=w441, "layout options"=w440, "report type (Quick Print)"=w439, "VI path"=w438) -> ()  [unwired: 6 in, 2 out]
      }
      frame "Email" {
        w457 = "Roofing@cppwind.com"  # return address
        w454 = string[] ["kgompertz@cppwind.com"]  # Recipients
        n204 = local read "print?"() -> (w459:bool)
        n205 = Temporary Directory() -> (w447:path)
        n206 = Build Path(base path=w447, name or relative path="RoofSettings.png") -> (appended path=w448:path)
        n207 = Current VI's Path() -> (path=w458:path)
        n208 = call "Save PNG Image of Front Panel.vi"("VI Path"=w458, "File Path In"=w448) -> ("error out"=w453:errorcluster, "File Path Out"=w446:path)  [unwired: 8 in]
        n209 = case shown="True" w459 {
          tunnel: ["Recipients" w468] -> w456
          tunnel: [w464 w467] -> w460
          tunnel: [w463 w466] -> w462
          frame False {
            w463 = "Here are the requested Roof settings: "  # message
            w464 = "Roof Settings"  # subject
          }
          frame True {
            w466 = "Someone has printed these Roof settings:"  # message
            w467 = "RoofSettingsPrinted"  # subject
            w468 = string[] []  # Recipients
          }
        }
        n210 = Bundle By Name(cluster=T6 {"path"=path "", "data"="", "binary"=TRUE, "MIME content-type \n(application/octet-stream)"="application/octet-stream"}, "MIME content-type \n(application/octet-stream)"="image/png" ("MIME content-type \n(application/octet-stream)"), "path"=w446) -> (w450:T6)
        n211 = Build Array (concatenate)(w456, w454) -> (w455:string[])
        n212 = Build Array(w450) -> (w451:T22)
        n213 = call <vilib>:"SMTP Email Send Multiple Attachments.vi"("recipients"=w455, "mail server"="mail server", "return address"=w457, "subject ([No Subject])"=w460, "message"=w462, "attachments"=w451, "error in (no error)"=w453) -> ("invalid recipients"=→"Failed recipients":string[])  [unwired: 7 in, 1 out]
      }
      frame "CleanUp" {
        w471 = FALSE  # print?
        n214 = local write "print?"(w471) -> ()
        n215 = local write "email?"(w471) -> ()
        n216 = property on="Tab Control" class="TabCtl (strict)"("Val(Sgnl)"=T1."Print" ("Value (Signaling)")) -> ()  [unwired: 2 in, 2 out]
      }
      frame "Save Channel Names" {
        n217 = stacked-sequence {
          seq-local: [w479 _ _] -> [_ w505 _]
          seq-local: [_ w504 _] -> [_ _ w518]
          tunnel: w477 -> [_ _ w519]
          tunnel: w476 -> [_ _ w516]
          frame #0 {
            n218 = for {
              N: 3 -> [_]
              shift-right: [w487] -> w479
              shift-left: string[][] [] -> [w489]
              i -> [w483]
              n219 = Add(x=w483, y=4) -> (x+y=w484:i32)
              n220 = Increment(x=w483) -> (x+1=w481:i32)
              n221 = case shown="1, Default" w481 {
                tunnel: [w499 w500 w502] -> w492
                tunnel: [w498 w501 w503] -> w485
                frame 1, Default {
                  n222 = local read "Selector 4"() -> (w499:i32[])
                  n223 = property on="Selector 4" class="LstBox (strict)"() -> ("Item Names"=w498:string[])  [unwired: 2 in, 2 out]
                }
                frame 2 {
                  n224 = property on="Selector 5" class="LstBox (strict)"() -> ("Item Names"=w501:string[])  [unwired: 2 in, 2 out]
                  n225 = local read "Selector 5"() -> (w500:i32[])
                }
                frame 3 {
                  n226 = local read "Selector 6"() -> (w502:i32[])
                  n227 = property on="Selector 6" class="LstBox (strict)"() -> ("Item Names"=w503:string[])  [unwired: 2 in, 2 out]
                }
              }
              n228 = Format Into String(format string="%d" ("Format String"), initial string="Selector ", w484) -> (resulting string=w488:string)  [unwired: 1 in, 1 out]
              n229 = for {
                tunnel: w492 -> [w497] mode=indexing
                tunnel: w488 -> [w496]
                tunnel: [w494] -> w486 mode=indexing
                tunnel: w485 -> [w493]
                n230 = Index Array(array=w493, index=w497) -> (element=w495:string)
                n231 = Build Array(w496, w495) -> (w494:string[])
              }
              n232 = Build Array (concatenate)(w489, w486) -> (w487:string[][])
            }
          }
          frame #1 {
            n233 = local read "Search 4"() -> (w506:string)
            n234 = local read "Search 5"() -> (w507:string)
            n235 = local read "Search 6"() -> (w508:string)
            n236 = Build Array("Search 4 string" ("element"), w506) -> (w512:string[])
            n237 = Build Array("Search 6 string" ("element"), w508) -> (w514:string[])
            n238 = Build Array("Search 5 string" ("element"), w507) -> (w513:string[])
            n239 = Build Array (concatenate)(w505, w512, w513, w514) -> (w504:string[][])
          }
          frame #2 {
            n240 = call "Setup_Filepath.vi"("Setup File Type"=Setup_Filetype."General", "Filename in"=w516) -> ("Filename Out"=w515:path)  [unwired: 1 out]
            n241 = Array Size(array=w518) -> (size(s)=w522:i32[])
            n242 = Index Array(array=w522, index=1 ("Index")) -> (element=w521:i32)
            n243 = Not Equal To 0?(x=w521) -> (x != 0?=w520:bool)
            n244 = case shown="True" w520 {
              tunnel: w515 -> [w524 w529]
              tunnel: w518 -> [_ w530]
              tunnel: w519 -> [_ w531]
              frame False {
                n245 = Delete(path (use dialog)=w524) -> ()  [unwired: 1 in, 6 out]
              }
              frame True {
                w525 = FALSE  # append to file? (new file:F)
                n246 = call "Ch_names_to_rows.vi"("Channel Names"=w531) -> ("3 Row names"=w532:string[][])
                n247 = Build Array (concatenate)(w532, w530) -> (w527:string[][])
                n248 = Array To Spreadsheet String(array=w527, 3:"%s" ("format string")) -> (spreadsheet string=w526:string)  [unwired: 1 out]
                n249 = call "Write_File_Simple.vi"("append to file? (new file:F)"=w525, "character string"=w526, "file path"=w529) -> ()  [unwired: 2 out]
              }
            }
          }
        }
        n250 = local read "stop"() -> (w474:bool)
        n251 = Not(x=w474) -> (.not. x?=w473:bool)
      }
    }
  }
